vi "acquire.vi"(9 "Samples per acquisition":i32, 11 "Sampling rate(samples/sec)":dbl) -> ()   [LabVIEW 2014]
panel:
  out "Output":cluster{i32, i32, dbl[]}(graph)
  in  "?":bool
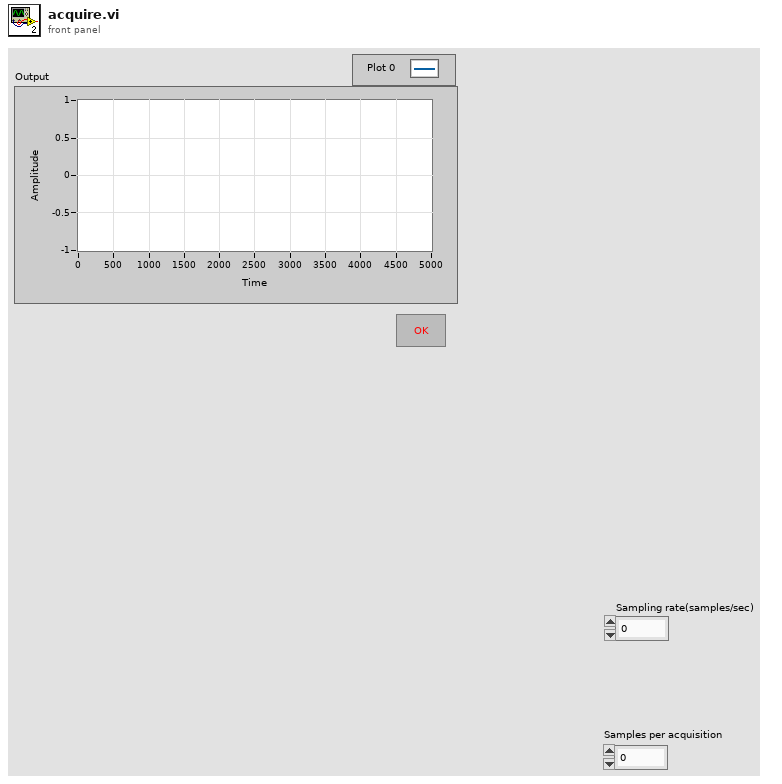
[diagram p1: front panel]
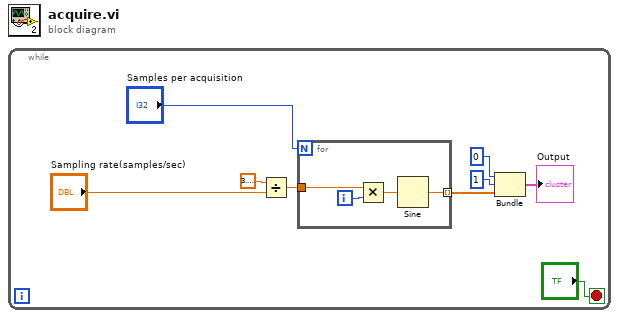
[diagram p0: block diagram]
diagram:
  n1 = while {
    stop <- "?" stop-if-true
    n2 = Divide(x=3.141592653589793, y="Sampling rate(samples/sec)") -> (x/y=w8:dbl)
    n3 = for {
      N: "Samples per acquisition" -> [_]
      tunnel: w8 -> [w13]
      tunnel: [w10] -> w7 mode=indexing
      i -> [w12]
      n4 = Multiply(x=w13, y=w12) -> (x*y=w11:dbl)
      n5 = Sine(x=w11) -> (sin(x)=w10:dbl)
    }
    n6 = Bundle(0, 1, w7) -> (→"Output":cluster{i32, i32, dbl[]})  [unwired: 1 in]
  }
